vi "Clear Error.vi"(5 "Error Name":string[](array[string]), 7 "Error Scope":string[](array[string]), 8 "Error In":errorcluster, 11 "Error Source":string[](array[string])) -> (0 "Error Out":errorcluster)   [LabVIEW 2016, in "Stream Error.lvlib"]
doc: "--\nCopyright © 2017 Composed SystemsI All rights reserved.\n\nAuthor: Jon McBee <jon.mcbee@composed.io>\n\nThis library is provided \"AS IS\" ,WITHOUT WARRANTIES OR\nCONDITIONS OF ANY KIND, either express or implied.\n\nComposed Systems -- composed.io\n\nStream 0.0.1.1\nJon McBee - Composed Systems\nCopyright (c) 2017, Composed Systems"
uses:
  <userlib>/Composed Systems/Stream/Error/Stream Error.lvlib
  <userlib>/Composed Systems/Stream/Error/Classes/Error Interface/Error UID.ctl
  <userlib>/Composed Systems/Stream/Error/Classes/Error Interface/Error Interface.lvclass
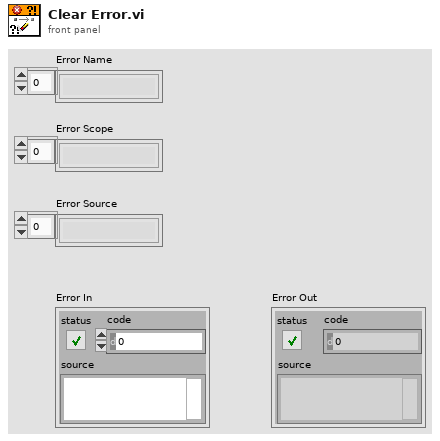
[diagram p1: front panel]
types:
  T1 = typedef "Stream Error.lvlib/Error Interface.lvclass/Error UID.ctl" = u16
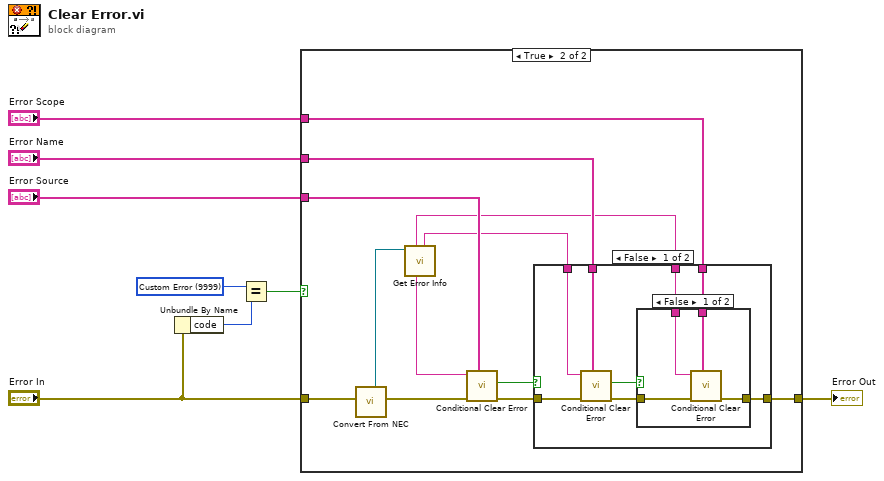
[diagram p0: block diagram]
diagram:
  w7 = T1 9999 items=["Custom Error"=9999] ("Custom Error Codes")
  n1 = Unbundle By Name("Error In") -> ("code"=w8:i32)
  n2 = Equal?(x=w7, y=w8) -> (x = y?=w6:bool)
  n3 = case shown="True" w6 {
    tunnel: "Error In" -> [w9 w21]
    tunnel: [w9 w12] -> w4
    tunnel: "Error Name" -> [_ w15]
    tunnel: "Error Source" -> [_ w18]
    tunnel: "Error Scope" -> [_ w14]
    frame False {
    }
    frame True {
      n4 = call <userlib>:"Convert From NEC.vi"("error in (no error)"=w21) -> ("error out"=w19:errorcluster, "Error Interface out"=w20:refnum<class "Error Interface.lvclass">)  [unwired: 9 in]
      n5 = call-dynamic "Get Error Info.vi"("Error Interface in"=w20) -> ("Error Name"=w13:string, "Error Source"=w17:string, "Error Scope"=w11:string)  [unwired: 6 in, 2 out]
      n6 = call <userlib>:"Conditional Clear Error.vi"("String Array"=w18, "error in (no error)"=w19, "Search String"=w17) -> ("error out"=w16:errorcluster, "Error Cleared?"=w10:bool)  [unwired: 7 in]
      n7 = case shown="False" w10 {
        tunnel: w16 -> [w29 w35]
        tunnel: w15 -> [w28 _]
        tunnel: w14 -> [w27 _]
        tunnel: w13 -> [w26 _]
        tunnel: [w24 w35] -> w12
        tunnel: w11 -> [w23 _]
        frame False {
          n8 = call <userlib>:"Conditional Clear Error.vi"("String Array"=w28, "error in (no error)"=w29, "Search String"=w26) -> ("error out"=w25:errorcluster, "Error Cleared?"=w22:bool)  [unwired: 7 in]
          n9 = case shown="False" w22 {
            tunnel: w27 -> [w33 _]
            tunnel: w25 -> [w32 w34]
            tunnel: [w31 w34] -> w24
            tunnel: w23 -> [w30 _]
            frame False {
              n10 = call <userlib>:"Conditional Clear Error.vi"("String Array"=w33, "error in (no error)"=w32, "Search String"=w30) -> ("error out"=w31:errorcluster)  [unwired: 7 in, 1 out]
            }
            frame True {
            }
          }
        }
        frame True {
        }
      }
    }
  }
  "Error Out" <- w4
